vi "ErrorHandling_GetError.vi"(8 "Fehler (Eingang, kein Fehler)":errorcluster caption="Error_In", 11 "Referenz_In":refnum<visa-resource-name>) -> (0 "Fehler (Ausgang)":errorcluster caption="Error_Out", 1 "communication_data":T1, 2 "Next Error":string, 3 "Referenz_Out":refnum<visa-resource-name>)   [LabVIEW 2018, in "OXYGEN.lvlib"]
doc: "Queries the next element in the Error Queue"
uses:
  OXYGEN.lvlib
  TypeDefs/Cluster_RawCommData.ctl
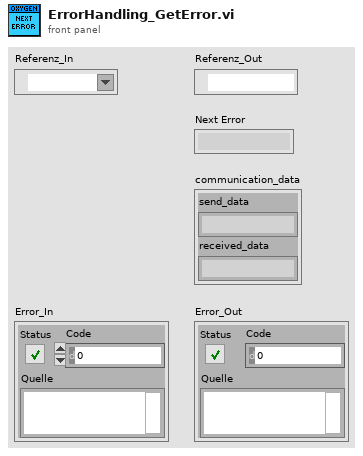
[diagram p1: front panel]
types:
  T1 = typedef "OXYGEN.lvlib/Cluster_RawCommData.ctl" = cluster{"send_data":string, "received_data":string}
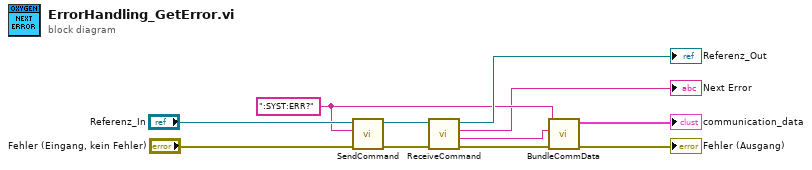
[diagram p0: block diagram]
diagram:
  w5 = ":SYST:ERR?" ("Schreibpuffer")
  n1 = call "SendCommand.vi"("error in (no error)"="Fehler (Eingang, kein Fehler)", "String to Send"=w5, "OXY_SCPI Reseource In"="Referenz_In") -> ("error out"=w7:errorcluster, "OXY_SCPI Reseource Out"=w6:refnum<visa-resource-name>)  [unwired: 7 in]
  n2 = call "ReceiveCommand.vi"("error in (no error)"=w7, "OXY_SCPI Reseource In"=w6) -> ("error out"=w2:errorcluster, "received Data with Header"=w4:string, "received Data"=→"Next Error":string, "OXY_SCPI Reseource Out"=→"Referenz_Out":refnum<visa-resource-name>)  [unwired: 6 in]
  n3 = call "BundleCommData.vi"("error in (no error)"=w2, "received_data"=w4, "send_data"=w5) -> ("error out"=→"Fehler (Ausgang)":errorcluster, "communication_data"=→"communication_data":T1)  [unwired: 7 in]
